vi "4.4.vi"() -> ()   [LabVIEW 2017]
panel:
  in  "实时温度":dbl
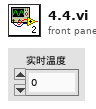
[diagram p1: front panel]
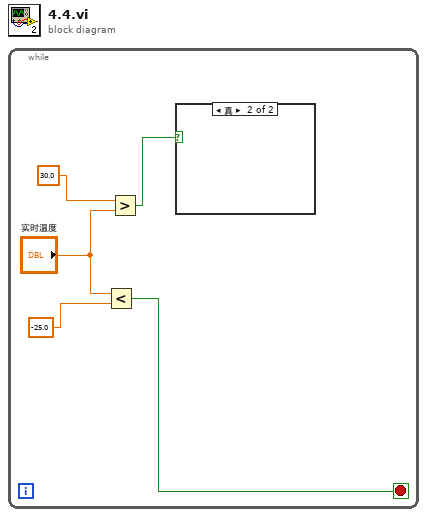
[diagram p0: block diagram]
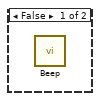
[diagram p2: hidden frame]
diagram:
  n1 = while {
    stop <- w2 stop-if-true
    n2 = Less?(x="实时温度", y=-25.0) -> (x < y?=w2:bool)
    n3 = Greater?(x=30.0, y="实时温度") -> (0:w3:bool)
    n4 = case shown="真" w3 {
      frame False {
        n5 = call <vilib>:"Beep.vi"() -> ()  [unwired: 12 in]
      }
      frame True {
      }
    }
  }
